vi "Port Close.vi"(8 "error in (no error)":errorcluster, 11 "MSX-E3711 in":refnum<class "MSX-E3711.lvclass">) -> (0 "error out":errorcluster, 3 "MSX-E3711 out":refnum<class "MSX-E3711.lvclass">)   [LabVIEW 2014, in "MSX-E3711.lvlib" / "MSX-E3711.lvclass"]
uses:
  MSX-E3711.lvclass
  MSX-E3711.lvclass/MSX-E3711.ctl
  API/MSX-E3711_dll.lvlib
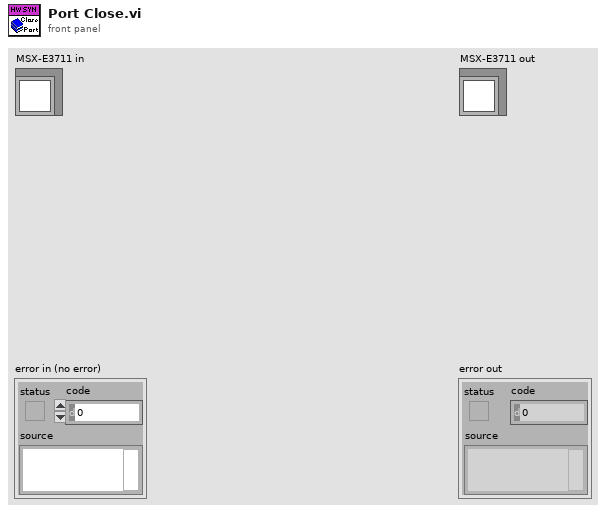
[diagram p1: front panel]
types:
  T1 = typedef "MSX-E3711_dll.lvlib/Connection Data.ctl" = cluster{"MX371x refnum":refnum<k24>, "IP":string, "Connection ID ":refnum<k5>, "MXCommon refnum":refnum<k24>}
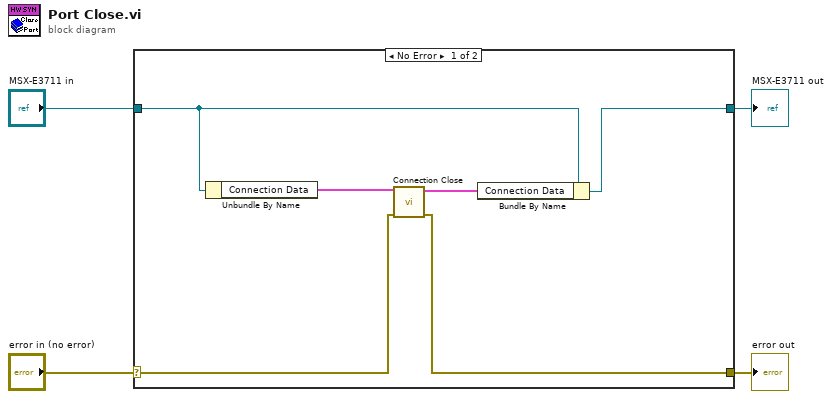
[diagram p0: block diagram]
diagram:
  n1 = case shown="No Error" "error in (no error)" {
    selector: "error in (no error)" -> [w9 w12]
    tunnel: [w8 w12] -> w3
    tunnel: [w6 w11] -> w1
    tunnel: "MSX-E3711 in" -> [w7 w11]
    frame No Error {
      n2 = Unbundle By Name(w7) -> ("Connection Data"=w10:T1)
      n3 = call "Connection Close.vi"("error in (no error)"=w9, "Connection Data In"=w10) -> ("error out"=w8:errorcluster, "Connection Data Out"=w5:T1)  [unwired: 8 in]
      n4 = Bundle By Name(cluster=w7, "Connection Data"=w5) -> (w6:refnum<class "MSX-E3711.lvclass">)
    }
    frame Error {
    }
  }
  "error out" <- w3
  "MSX-E3711 out" <- w1
